vi "filtro passa basso.vi"(9 "sampling freq: fs":dbl, 10 "Cluster":T1, 11 "Waveform":waveform(dbl)) -> (2 "Waveform 2":waveform(dbl))   [LabVIEW 2016]
uses:
  <vilib>/Analysis/3filter.llb/Filter Passband Type.ctl
  <vilib>/Analysis/3filter.llb/Butterworth Filter (DBL).vi
  <vilib>/Analysis/NI_AALBase.lvlib
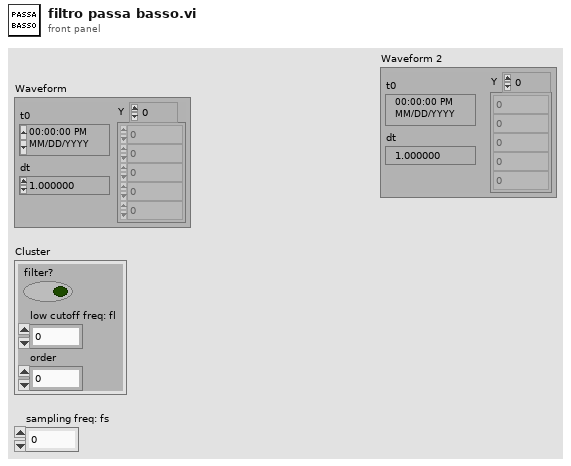
[diagram p1: front panel]
types:
  T1 = cluster{"filter?":bool, "low cutoff freq: fl":dbl, "order":i32}
  T2 = typedef "NI_AALBase.lvlib/Filter Passband Type.ctl" = enum32{"Lowpass", "Highpass", "Bandpass", "Bandstop"}
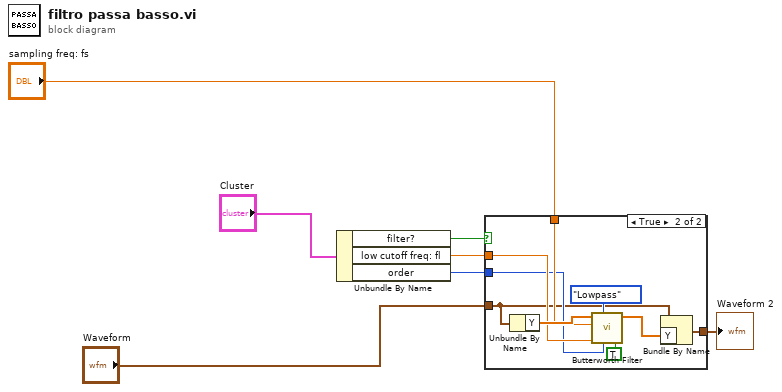
[diagram p0: block diagram]
diagram:
  n1 = Unbundle By Name("Cluster") -> ("filter?"=w4:bool, "low cutoff freq: fl"=w5:dbl, "order"=w6:i32)
  n2 = case shown="True" w4 {
    tunnel: "Waveform" -> [w8 w9]
    tunnel: [w8 w15] -> w1
    tunnel: "sampling freq: fs" -> [_ w13]
    tunnel: w5 -> [_ w12]
    tunnel: w6 -> [_ w11]
    frame False {
    }
    frame True {
      n3 = Unbundle By Name(w9) -> ("Y"=w16:dbl[])
      n4 = call-poly <vilib>:"Butterworth Filter.vi"("init/cont (init:F)"=TRUE, "order"=w11, "filter type"=Filter_Passband_Type."Lowpass", "low cutoff freq: fl"=w12, "sampling freq: fs"=w13, "X"=w16) -> ("Filtered X"=w17:dbl[])  [unwired: 2 in, 1 out]
      n5 = Bundle By Name(cluster=w9, "Y"=w17) -> (w15:waveform(dbl))
    }
  }
  "Waveform 2" <- w1
